vi "Remove IntelliSense Control.vi"(0 "IntelliSenseStringControl":refnum<class "IntelliSenseStringControl.lvclass">) -> (1 "IntelliSenseStringControl":refnum<class "IntelliSenseStringControl.lvclass">, 3 "removed?":bool)   [LabVIEW 2016, in "StringIntelliSense.lvlib" / "IntelliSenseStringControl.lvclass"]
uses:
  IntelliSenseStringControl.lvclass
  StringMonitorUserData.vi
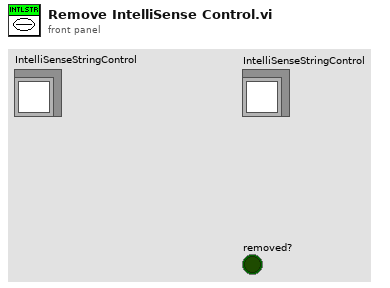
[diagram p1: front panel]
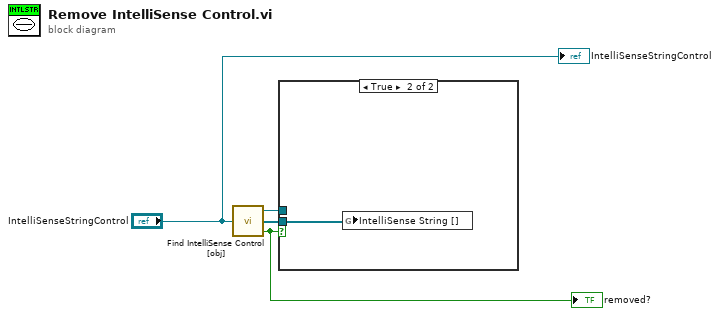
[diagram p0: block diagram]
diagram:
  n1 = call "Find IntelliSense Control [obj].vi"("IntelliSenseStringControl"="IntelliSenseStringControl") -> ("Found IntelliSenseStringControl"=w3:refnum<class "IntelliSenseStringControl.lvclass">, "Other IntelliSense String []"=w4:refnum<class "IntelliSenseStringControl.lvclass">[], "Found?"=w2:bool)
  "removed?" <- w2
  n2 = case shown="True" w2 {
    tunnel: w4 -> [_ w5]
    tunnel: w3 -> [_ _]
    frame False {
    }
    frame True {
      n3 = global write "StringMonitorUserData.vi" "IntelliSense String []"(w5) -> ()
    }
  }
  "IntelliSenseStringControl" <- "IntelliSenseStringControl"
